vi "Query Multi Eval Meas Modulation Extreme Limit Check Results.vi"(8 "error in (no error)":errorcluster, 10 "Instance (1)":T1=1, 11 "VISA resource name":refnum<visa-resource-name>) -> (0 "error out":errorcluster, 1 "Limit Check Results":i32[](array[numeric]), 2 "Reliability":i32, 3 "VISA resource name out":refnum<visa-resource-name>, 5 "Out Of Tolerance":i32)   [LabVIEW 2020, in "Rohde&Schwarz CMWXP NR FR1 Measurement.lvlib"]
doc: "Return the extreme single value limit check results.\n\nAttribute:\nRSCMWXPNRFR1M_ATTR_QUERY_MULTI_EVAL_MEAS_MODULATION_EXTREME_LIMIT_CHECK_RESULTS\n\nRemote-control command:\nCALCulate:NRSub:MEAS<i>:MEValuation:MODulation:EXTReme?"
uses:
  <instrlib>/Rohde&Schwarz CMWXP NR FR1 Measurement/Rohde&Schwarz CMWXP NR FR1 Measurement.lvlib
  <instrlib>/Rohde&Schwarz CMWXP NR FR1 Measurement/Private/_Instance.ctl
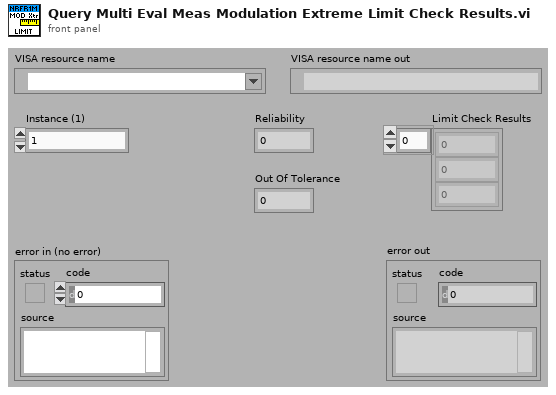
[diagram p1: front panel]
types:
  T1 = typedef "Rohde&Schwarz CMWXP NR FR1 Measurement.lvlib/_Instance.ctl" = i32
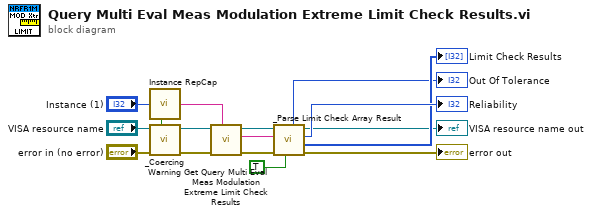
[diagram p0: block diagram]
diagram:
  n1 = call <instrlib>:"Instance RepCap.vi"("Instance In"="Instance (1)") -> ("In Range?"=w13:bool, "RepCap Identifier Out"=w12:string)  [unwired: 1 in]
  n2 = call <instrlib>:"_Coercing Warning.vi"("In Range?"=w13, "error in (no error)"="error in (no error)", "VISA resource name"="VISA resource name") -> ("error out"=w10:errorcluster, "VISA resource name out"=w11:refnum<visa-resource-name>)  [unwired: 7 in]
  n3 = call "Get Query Multi Eval Meas Modulation Extreme Limit Check Results"("Repeated Capabilities"=w12, "error in (no error)"=w10, "instrument handle"=w11) -> ("error out"=w9:errorcluster, "Query Multi Eval Meas Modulation Extreme Limit Check Results"=w7:string, "instrument handle out"=w8:refnum<visa-resource-name>)  [unwired: 6 in]
  n4 = call <instrlib>:"_Parse Limit Check Array Result.vi"("error in (no error)"=w9, "Input String"=w7, "VISA resource name"=w8, "Out of tolerance? (F)"=TRUE) -> ("Out Of Tolerance"=→"Out Of Tolerance":i32, "error out"=→"error out":errorcluster, "Results"=→"Limit Check Results":i32[], "Reliability"=→"Reliability":i32, "VISA resource name out"=→"VISA resource name out":refnum<visa-resource-name>)  [unwired: 2 in]
